vi "Write Power FIFO.vi"(6 "FIFO Timestamps":T1, 8 "error in (no error)":errorcluster, 9 "Timeout (ms)":i32=100, 10 "Data In":T2[](array[typedef])=[{"measurement"=[], "dT"=0.0, "Timestamp"=0, "Read Lock"=FALSE}, {"measurement"=[], "dT"=0.0, "Timestamp"=0, "Read Lock"=FALSE}], 11 "CIFTag in":refnum<class "CIF_NIChn_Fifo_Power.lvclass">) -> (0 "error out":errorcluster, 1 "timed out?":bool, 2 "Data Out":T2[](array[typedef]), 3 "CIFTag out":refnum<class "CIF_NIChn_Fifo_Power.lvclass">)   [LabVIEW 2021, in "CIF_NIChn_Fifo_Power.lvclass"]
uses:
  CIF_NIChn_Fifo_Power.lvclass
  CIF_NIChn_Fifo_Power.lvclass/CIF_NIChn_Fifo_Power.ctl
  NIChn/CIF_NIChn.lvclass
  <vilib>/CIFChannels/CIFChannelCore.lvlib
  D:/dev/Packages/Channel_Manager/src/CIF_NIChn/NIChn/CIF_NIChn.lvclass
  ChannelCommon/typedef/Datatype Waveform.ctl
  ChannelCommon/ChannelCommon.lvlib
  ChannelCommon/typedef/TimeStamps.ctl
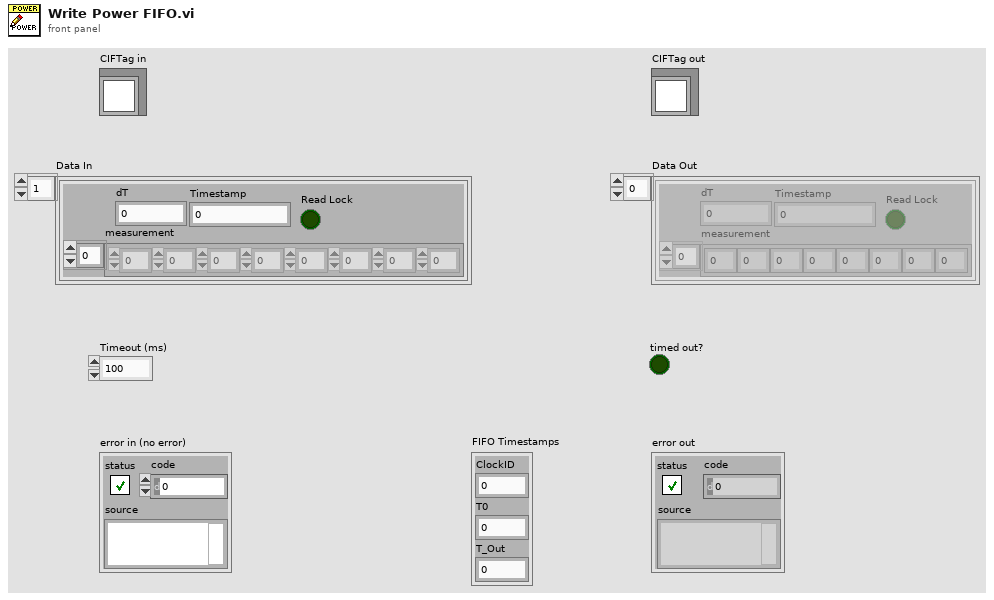
[diagram p1: front panel]
types:
  T1 = typedef "ChannelCommon.lvlib/TimeStamps.ctl" = cluster{"ClockID":u8, "T0":i64, "T_Out":i64}
  T2 = typedef "ChannelCommon.lvlib/Datatype Waveform.ctl" = cluster{"measurement":dbl[], "dT":dbl, "Timestamp":i64, "Read Lock":bool}
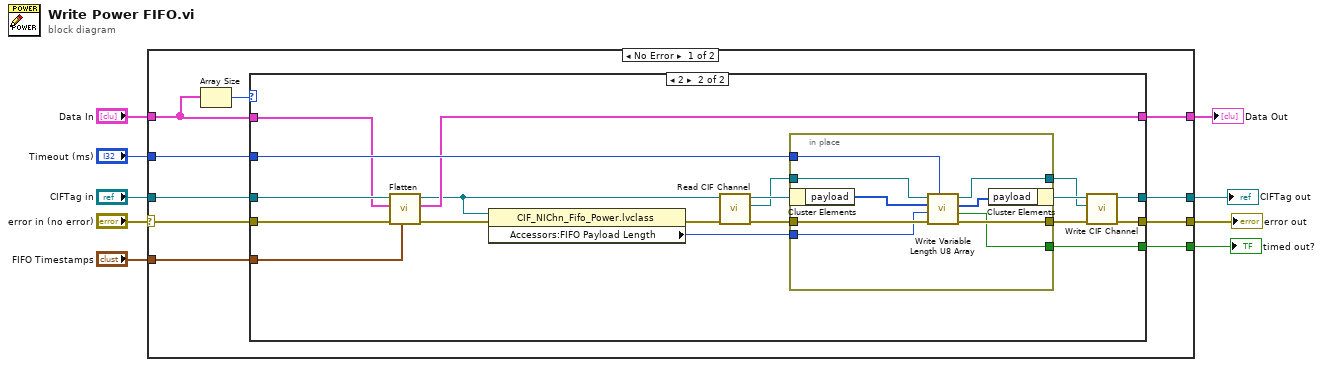
[diagram p0: block diagram]
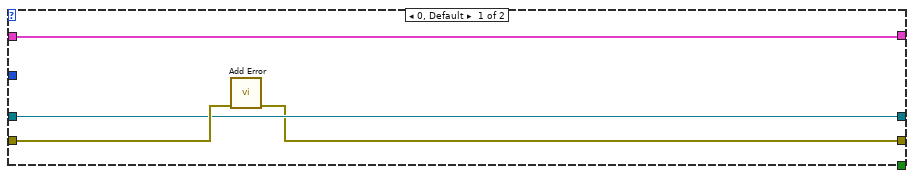
[diagram p2: hidden frame]
diagram:
  n1 = case shown="No Error" "error in (no error)" {
    selector: "error in (no error)" -> [w14 w54]
    tunnel: [w16 w54] -> w8
    tunnel: [w18 w53] -> w6
    tunnel: "CIFTag in" -> [w15 w53]
    tunnel: [w19 _] -> w5
    tunnel: "Timeout (ms)" -> [w17 _]
    tunnel: [w13 w52] -> w3
    tunnel: "Data In" -> [w12 w52]
    tunnel: "FIFO Timestamps" -> [w10 _]
    frame No Error {
      n2 = Array Size(array=w12) -> (size(s)=w11:i32)
      n3 = case shown="2" w11 {
        tunnel: [_ w42] -> w19
        tunnel: [w22 w38] -> w18
        tunnel: w17 -> [_ w34]
        tunnel: [w21 w33] -> w16
        tunnel: w15 -> [w22 w31]
        tunnel: w14 -> [w23 w29]
        tunnel: [w20 w27] -> w13
        tunnel: w12 -> [w20 w26]
        tunnel: w10 -> [_ w25]
        frame 0, Default {
          n4 = call "Add Error.vi"("error in (no error)"=w23) -> ("error out"=w21:errorcluster)  [unwired: 10 in]
        }
        frame 2 {
          n5 = call "Flatten.vi"("FIFO Timestamps"=w25, "error in (no error)"=w29, "Data"=w26, "CIFTag in"=w31) -> ("error out"=w30:errorcluster, "Data out"=w27:T2[], "CIFTag out"=w24:refnum<class "CIF_NIChn_Fifo_Power.lvclass">)  [unwired: 5 in]
          n6 = property class="CIF_NIChn_Fifo_Power.lvclass"(reference=w24, error in=w30) -> (error out=w32:errorcluster, "Accessors:FIFO Payload Length"=w28:u64)  [unwired: 1 out]
          n7 = call "Read CIF Channel.vi"("error in (no error)"=w32, "CIFTag in"=w24) -> ("error out"=w40:errorcluster, "CIF Channel"=w36:refnum<k21>, "CIFTag out"=w41:refnum<class "CIF_NIChn_Fifo_Power.lvclass">)  [unwired: 7 in]
          n8 = in-place {
            in-place-border: w40 -> [w51]
            in-place-border: [w50] -> w37
            in-place-border: [w49] -> w42
            in-place-border: w36 -> [w48]
            in-place-border: [w47] -> w35
            in-place-border: w34 -> [w46]
            in-place-border: w28 -> [w44]
            n9 = in-place-cluster #1(w41) -> ("payload"=w45:u8[])
            n10 = call <vilib>:"Write Variable Length U8 Array.vi"("Timeout (ms)"=w46, "error in"=w51, "numElements"=w44, "U8 Array in"=w45, "CIF Channel in"=w48) -> ("error out"=w50:errorcluster, "Timed out?"=w49:bool, "U8 Array out"=w43:u8[], "CIF Channel out"=w47:refnum<k21>)  [unwired: 3 in]
            n11 = in-place-cluster #1("payload"=w43) -> (w39:refnum<class "CIF_NIChn_Fifo_Power.lvclass">)
          }
          n12 = call "Write CIF Channel.vi"("error in (no error)"=w37, "CIF Channel"=w35, "CIFTag in"=w39) -> ("error out"=w33:errorcluster, "CIFTag out"=w38:refnum<class "CIF_NIChn_Fifo_Power.lvclass">)  [unwired: 7 in]
        }
      }
    }
    frame Error {
    }
  }
  "error out" <- w8
  "CIFTag out" <- w6
  "timed out?" <- w5
  "Data Out" <- w3
